vi "VisionAlign.vi"(11 "JoystickSpeed":dbl) -> (1 "Y":dbl, 2 "X":dbl, 3 "Z":dbl)   [LabVIEW 2018]
uses:
  <vilib>/Rock Robotics/Network Tables/NT Read Numeric Array.vi
  <vilib>/addons/control/pid/pid.llb/PID (DBL).vi
  Swerve/SwerveGlobals.vi
  <vilib>/Rock Robotics/Network Tables/NT Read Number.vi
  <vilib>/addons/control/pid/NI_PID_pid.lvlib
panel:
  out "MillisecondsToProcess":timestamp
  in  "AngleError":dbl=5.0
  in  "Distance PID":T1={"proportional gain (Kc)"=1.0, "integral time (Ti, min)"=0.01, "derivative time (Td, min)"=0.0} {"derivative time (Td, min)" format="%.3f"; "integral time (Ti, min)" format="%.3f"; "proportional gain (Kc)" format="%.3f"}
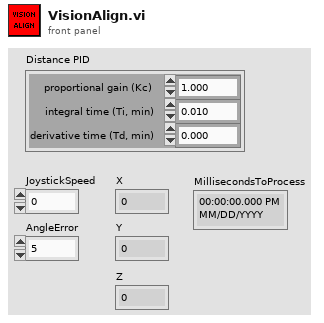
[diagram p1: front panel]
types:
  T1 = cluster{"proportional gain (Kc)":dbl, "integral time (Ti, min)":dbl, "derivative time (Td, min)":dbl}
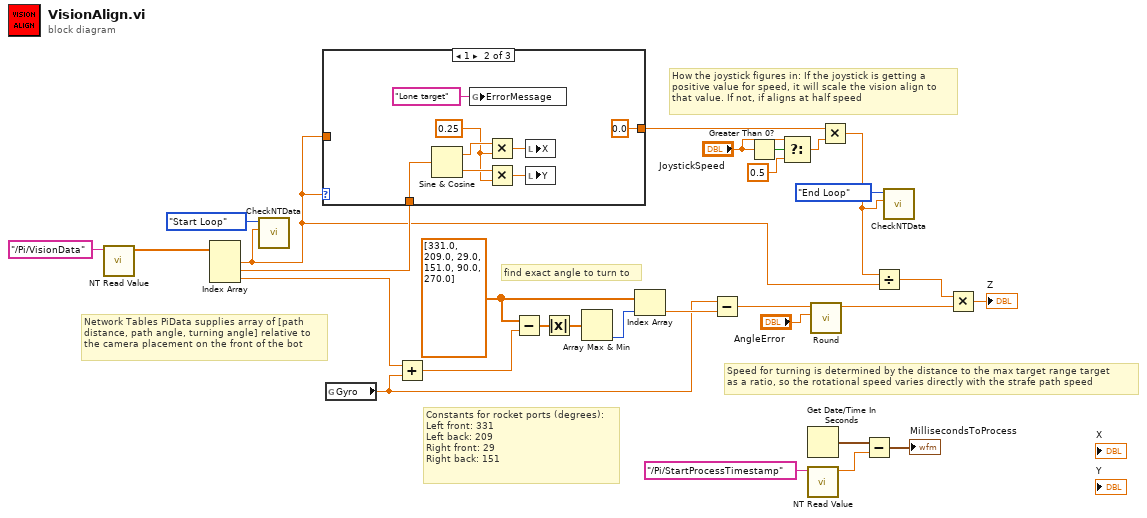
[diagram p0: block diagram]
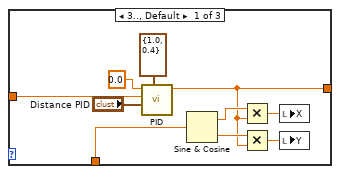
[diagram p2: hidden frame]
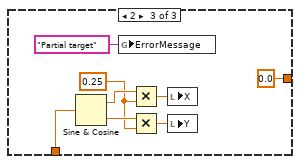
[diagram p3: hidden frame]
diagram:
  w19 = dbl[] [331.0, 209.0, 29.0, 151.0, 90.0, 270.0]
  # "find exact angle to turn to"
  # "How the joystick figures in: If the joystick is getting a\npositive value for speed, it will scale the vision align to\nthat value. If not, if aligns at half speed"
  # "Speed for turning is determined by the distance to the max target range target\nas a ratio, so the rotational speed varies directly with the strafe path speed"
  # "Constants for rocket ports (degrees):\nLeft front: 331\nLeft back: 209\nRight front: 29\nRight back: 151"
  # "Network Tables PiData supplies array of [path\ndistance, path angle, turning angle] relative to\nthe camera placement on the front of the bot"
  n1 = call-poly <vilib>:"NT Read Value.vi"("Name"="/Pi/VisionData" ("Client Name")) -> ("Numeric Array"=w5:dbl[])  [unwired: 9 in, 1 out]
  n2 = Index Array(array=w5) -> (element #1=w1:dbl, element #2=w17:dbl, element #3=w16:dbl)  [unwired: 3 in]
  n3 = call "CheckNTData.vi"("ValToCheck"=w1, "Mode"=enum16{"Start Loop", "End Loop"}."Start Loop") -> ()  [unwired: 10 in]
  n4 = case shown="1" w1 {
    tunnel: [w30 0.0 ("output") 0.0 ("output")] -> w24
    tunnel: w1 -> [w37 _ _]
    tunnel: w17 -> [w31 w43 w51]
    frame 3.., Default {
      n5 = call-poly <vilib>:"PID.vi"("output range"=cluster{"output high":dbl, "output low":dbl} {"output high"=1.0, "output low"=0.4}, "PID gains"="Distance PID", "process variable"=w37, "setpoint"=0.0) -> ("output"=w30:dbl)  [unwired: 6 in, 1 out]
      n6 = Sine & Cosine(0:w31) -> (1:w32:dbl, 2:w33:dbl)
      n7 = Multiply(x=w32, y=w30) -> (x*y=w35:dbl)
      n8 = Multiply(x=w33, y=w30) -> (x*y=w34:dbl)
      n9 = local write "X"(w35) -> ()
      n10 = local write "Y"(w34) -> ()
    }
    frame 1 {
      w42 = 0.25 ("y")
      n11 = Sine & Cosine(0:w43) -> (1:w45:dbl, 2:w46:dbl)
      n12 = global write "SwerveGlobals.vi" "ErrorMessage"("Lone target" ("ErrorMessage")) -> ()
      n13 = Multiply(x=w45, y=w42) -> (x*y=w41:dbl)
      n14 = Multiply(x=w46, y=w42) -> (x*y=w40:dbl)
      n15 = local write "X"(w41) -> ()
      n16 = local write "Y"(w40) -> ()
    }
    frame 2 {
      w50 = 0.25 ("y")
      n17 = Sine & Cosine(0:w51) -> (1:w52:dbl, 2:w53:dbl)
      n18 = global write "SwerveGlobals.vi" "ErrorMessage"("Partial target" ("ErrorMessage")) -> ()
      n19 = Multiply(x=w52, y=w50) -> (x*y=w49:dbl)
      n20 = Multiply(x=w53, y=w50) -> (x*y=w48:dbl)
      n21 = local write "X"(w49) -> ()
      n22 = local write "Y"(w48) -> ()
    }
  }
  n23 = global read "SwerveGlobals.vi" "Gyro"() -> (w14:dbl)
  n24 = Add(x=w16, y=w14) -> (x+y=w18:dbl)
  n25 = Subtract(x=w19, y=w18) -> (x-y=w22:dbl[])
  n26 = Absolute Value(x=w22) -> (abs(x)=w21:dbl[])
  n27 = Array Max & Min(array=w21) -> (min index (indices)=w20:i32)  [unwired: 3 out]
  n28 = Index Array(array=w19, index=w20) -> (element=w15:dbl)
  n29 = Subtract(x=w14, y=w15) -> (x-y=w12:dbl)
  n30 = Greater Than 0?(x="JoystickSpeed") -> (x > 0?=w27:bool)
  n31 = Select(t="JoystickSpeed", s=w27, f=0.5) -> (s? t:f=w23:dbl)
  n32 = Get Date/Time In Seconds() -> (seconds since 1Jan1904=w8:timestamp)
  n33 = call-poly <vilib>:"NT Read Value.vi"("Name"="/Pi/StartProcessTimestamp" ("Client Name")) -> ("Numeric"=w7:dbl)  [unwired: 9 in, 1 out]
  n34 = call "Round.vi"("Val"="AngleError", "Step"=w12) -> ("Val'"=w11:dbl)  [unwired: 9 in]
  n35 = Multiply(x=w24, y=w23) -> (x*y=w3:dbl)
  n36 = Subtract(x=w8, y=w7) -> (x-y=→"MillisecondsToProcess":timestamp)
  n37 = Divide(x=w3, y=w1) -> (x/y=w10:dbl)
  n38 = call "CheckNTData.vi"("ValToCheck"=w3, "Mode"=enum16{"Start Loop", "End Loop"}."End Loop") -> ()  [unwired: 10 in]
  n39 = Multiply(x=w10, y=w11) -> (x*y=→"Z":dbl)
